vi "Read Robodolf Controller State message.vi"(8 "error in (no error)":errorcluster, 11 "Controller State in":refnum<class "Controller State.lvclass">) -> (0 "error out":errorcluster, 2 "Controller State":T1, 3 "Controller State out":refnum<class "Controller State.lvclass">)   [LabVIEW 2015, in "RDS Child Messages.lvlib" / "Controller State.lvclass"]
uses:
  Controller State.lvclass
  Actors/RDS Controller Actor/RDS Controller Actor/Controller.ctl
  Controller State.lvclass/Controller State.ctl
  Actors/RDS Controller Actor/RDS Controller Actor/RDS Controller Actor.lvlib
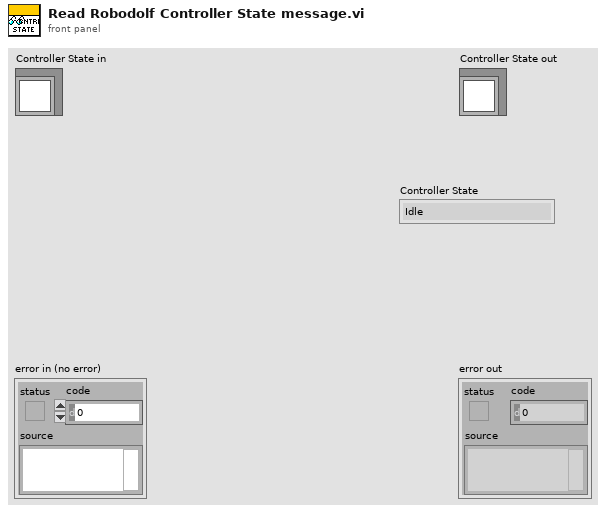
[diagram p1: front panel]
types:
  T1 = typedef "RDS Controller Actor.lvlib/Controller.ctl" = enum16{"Idle", "Local Remote Control", "Shore Remote Control", "Mission Control"}
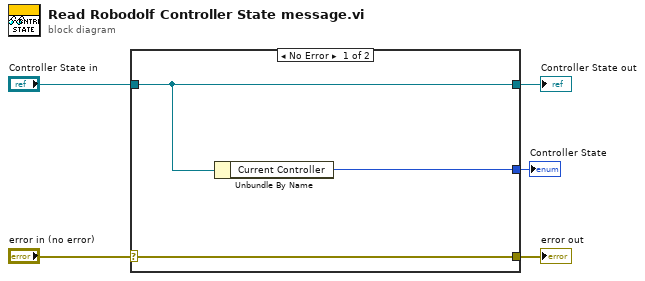
[diagram p0: block diagram]
diagram:
  n1 = case shown="No Error" "error in (no error)" {
    selector: "error in (no error)" -> [w8 w9]
    tunnel: [w8 w9] -> w4
    tunnel: [w7 w10] -> w2
    tunnel: "Controller State in" -> [w7 w10]
    tunnel: [w6 _] -> w1
    frame No Error {
      n2 = Unbundle By Name(w7) -> ("Current Controller"=w6:T1)
    }
    frame Error {
    }
  }
  "error out" <- w4
  "Controller State out" <- w2
  "Controller State" <- w1
